vi "IMD Test Settings Get Configuration Data as String.vi"(8 "error in":errorcluster, 10 "Configuration Name":string, 11 "IMD Test Settings in":refnum<class "IMD Test Settings.lvclass">) -> (0 "error out":errorcluster, 1 "2SG Frequency":string, 2 "SA Reference Level":string, 3 "IMD Test Settings out":refnum<class "IMD Test Settings.lvclass">, 4 "2SG Relative Power Level":string, 5 "SA Frequency Offset":string, 6 "2SG Waveform Name":string, 7 "SG Frequency Offset":string)   [LabVIEW 2016, in "IMD Test Settings.lvlib" / "IMD Test Settings.lvclass"]
uses:
  IMD Test Settings.lvclass
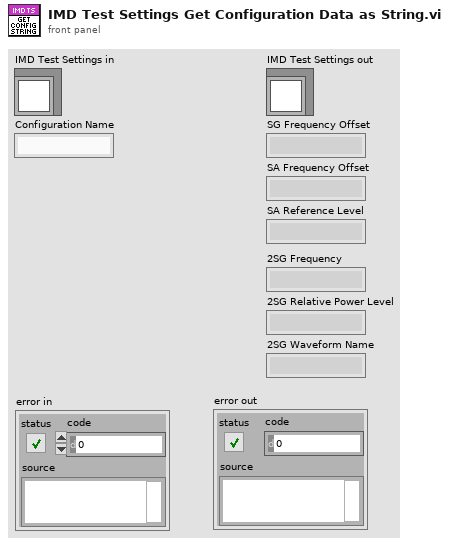
[diagram p1: front panel]
types:
  T1 = typedef "IMD Test Settings.lvlib/IMD Test Settings.lvclass/IMD Settings Cluster.ctl" = cluster{"SG Frequency Offset":dbl, "SA Frequency Offset":dbl, "SA Reference Level":dbl, "2SG Frequency":dbl, "2SG Relative Power Level":dbl, "2SG Waveform Name":string}
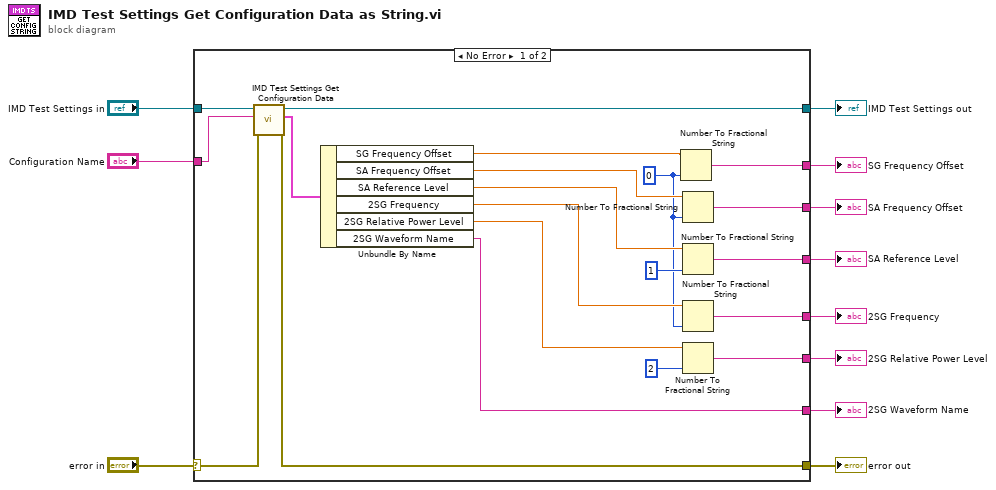
[diagram p0: block diagram]
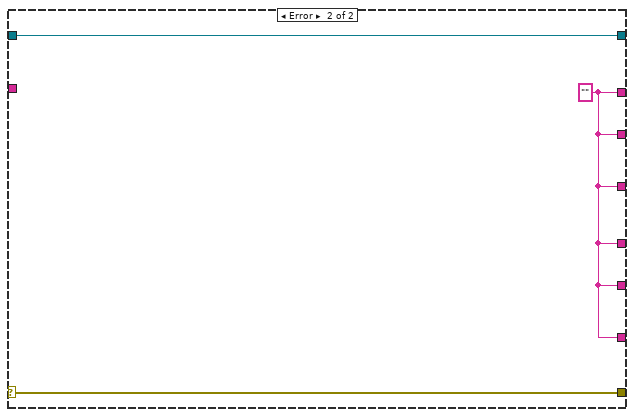
[diagram p2: hidden frame]
diagram:
  n1 = case shown="No Error" "error in" {
    selector: "error in" -> [w25 w34]
    tunnel: [w24 w34] -> w5
    tunnel: [w26 w33] -> w9
    tunnel: [w30 w32] -> w8
    tunnel: [w28 w32] -> w7
    tunnel: "Configuration Name" -> [w23 _]
    tunnel: "IMD Test Settings in" -> [w27 w33]
    tunnel: [w19 w32] -> w4
    tunnel: [w15 w32] -> w3
    tunnel: [w14 w32] -> w2
    tunnel: [w13 w32] -> w1
    frame No Error {
      w12 = i16 0 ("precision (6)")
      n2 = call "IMD Test Settings Get Configuration Data.vi"("error in"=w25, "Configuration Name"=w23, "IMD Test Settings in"=w27) -> ("error IO"=w24:errorcluster, "IMD Settings Cluster"=w22:T1, "IMD Test Settings out"=w26:refnum<class "IMD Test Settings.lvclass">)  [unwired: 6 in]
      n3 = Unbundle By Name(w22) -> ("SG Frequency Offset"=w31:dbl, "SA Frequency Offset"=w29:dbl, "SA Reference Level"=w20:dbl, "2SG Frequency"=w17:dbl, "2SG Relative Power Level"=w16:dbl, "2SG Waveform Name"=w15:string)
      n4 = Number To Fractional String(number=w31, precision (6)=w12) -> (F-format string=w30:string)  [unwired: 2 in]
      n5 = Number To Fractional String(number=w29, precision (6)=w12) -> (F-format string=w28:string)  [unwired: 2 in]
      n6 = Number To Fractional String(number=w20, precision (6)=i16 1) -> (F-format string=w19:string)  [unwired: 2 in]
      n7 = Number To Fractional String(number=w17, precision (6)=w12) -> (F-format string=w13:string)  [unwired: 2 in]
      n8 = Number To Fractional String(number=w16, precision (6)=i16 2) -> (F-format string=w14:string)  [unwired: 2 in]
    }
    frame Error {
      w32 = ""
    }
  }
  "IMD Test Settings out" <- w9
  "SG Frequency Offset" <- w8
  "SA Frequency Offset" <- w7
  "error out" <- w5
  "SA Reference Level" <- w4
  "2SG Frequency" <- w1
  "2SG Relative Power Level" <- w2
  "2SG Waveform Name" <- w3
